vi "ChkOrigDly.vi"(8 "错误输入（无错误）":errorcluster, 10 "Chan":u8, 11 "零位延时":u32) -> (0 "错误输出":errorcluster, 3 "返回值":i32)   [LabVIEW 2014]
uses:
  X86Dll/ZXUTConfigMgr.dll
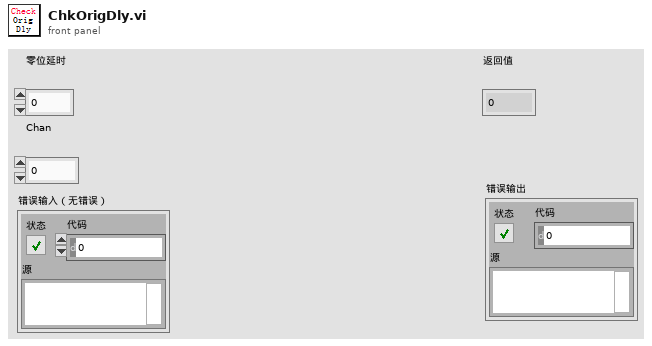
[diagram p1: front panel]
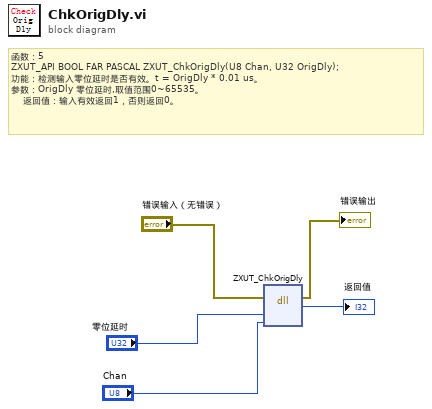
[diagram p0: block diagram]
diagram:
  # "函数：5\nZXUT_API BOOL\tFAR PASCAL ZXUT_ChkOrigDly(U8 Chan, U32 OrigDly);\n功能：检测输入零位延时是否有效。t = OrigDly * 0.01 us。\n参数：OrigDly 零位延时,取值范围0~65535。\n\t   返回值：输入有效返回1，否则返回0。"
  n1 = dll-call lib="D:/Software/Utrasonic on-line monitoring/X86Dll/ZXUTConfigMgr.dll" fn="ZXUT_ChkOrigDly"(error in="错误输入（无错误）", "OrigDly"="零位延时", "Chan"="Chan") -> (error out=→"错误输出":errorcluster, "返回值"=→"返回值":i32)  [unwired: 4 in, 1 out]
